vi "CmdexPwmShift.vi"(8 "Uart Input":cluster{u64} {"?" format="%x"}, 9 "Shift":sgl, 10 "PWM Id":enum16{"PWM0", "PWM1", "PWM2", "PWM3"}(ring), 11 "Error Input":errorcluster) -> (0 "Uart Output":cluster{u64} {"?" format="%x"}, 3 "Error Output":errorcluster)   [LabVIEW 2019]
doc: "<B>Cmdexs</B>\nChange phase-shift of the PWM."
uses:
  dll/LabViewUart.dll
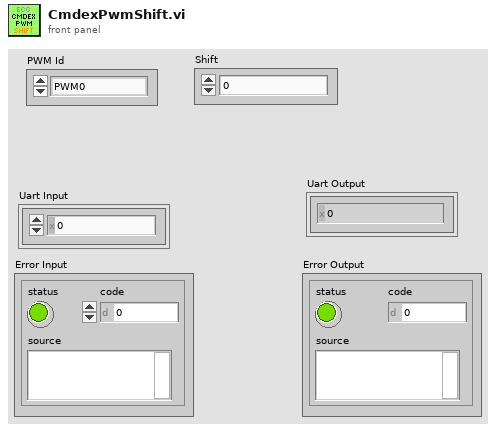
[diagram p1: front panel]
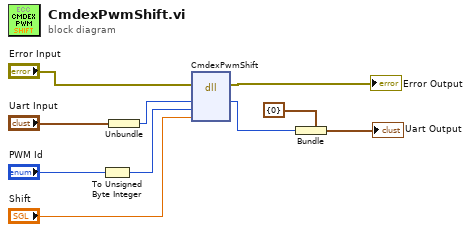
[diagram p0: block diagram]
diagram:
  n1 = To Unsigned Byte Integer(number="PWM Id") -> (unsigned 8bit integer=w5:u8)
  n2 = Unbundle("Uart Input") -> (w7:u64)
  n3 = dll-call lib="D:/Google Drive/INC-2020/INC352/INC352-2020/LabVIEW/examples/uart-cmdex/SubVI/dll/LabViewUart.dll" fn="CmdexPwmShift"(error in="Error Input", "Uart Handle"=w7, "id"=w5, "shift"="Shift") -> (error out=→"Error Output":errorcluster, "Uart Handle"=w2:u64)  [unwired: 5 in, 1 out]
  n4 = Bundle(cluster=cluster{u64} {0}, w2) -> (→"Uart Output":cluster{u64})
